vi "radians_to_degrees.vi"(1 "radians":dbl format="%.2f") -> (0 "degrees":dbl format="%.2f")   [LabVIEW 2010]
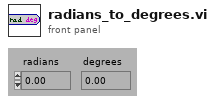
[diagram p1: front panel]
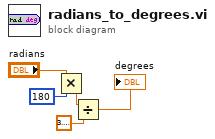
[diagram p0: block diagram]
diagram:
  n1 = Multiply(x="radians", y=180) -> (x*y=w4:dbl)
  n2 = Divide(x=w4, y=3.141592653589793) -> (x/y=→"degrees":dbl)
